vi "pinMode.vi"(3 "error in (no error)":errorcluster, 4 "Mode":enum32{"Output", "Input"}(ring), 5 "Terminal":u8, 6 "VISA Refnum in":refnum<visa-resource-name>) -> (0 "error out":errorcluster, 1 "pinMode":u8[](array[numeric]), 2 "VISA Refnum out":refnum<visa-resource-name>)   [LabVIEW 2016]
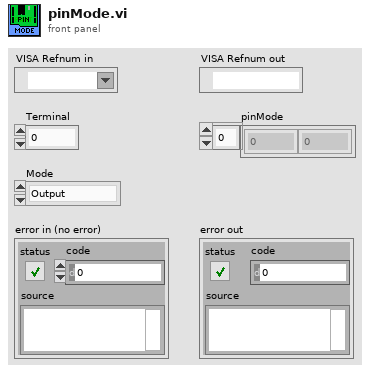
[diagram p1: front panel]
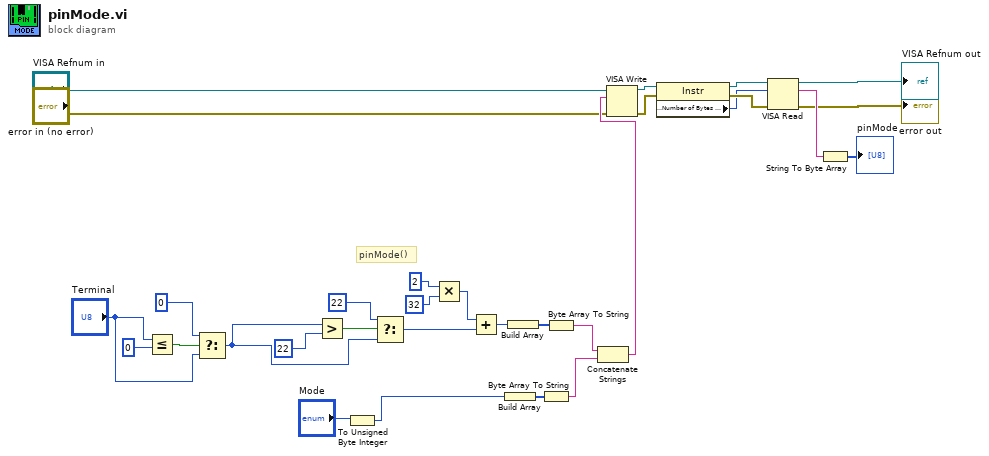
[diagram p0: block diagram]
diagram:
  # "pinMode()"
  n1 = Less Or Equal?(x="Terminal", y=u8 0) -> (x <= y?=w17:bool)
  n2 = Select(t=u8 0, s=w17, f="Terminal") -> (s? t:f=w20:u8)
  n3 = Greater?(x=w20, y=u8 22) -> (0:w12:bool)
  n4 = To Unsigned Byte Integer(number="Mode") -> (unsigned 8bit integer=w31:u8)
  n5 = Select(t=u8 22, s=w12, f=w20) -> (s? t:f=w29:u8)
  n6 = Multiply(x=u8 2, y=u8 32) -> (x*y=w15:u8)
  n7 = Add(x=w15, y=w29) -> (x+y=w21:u8)
  n8 = Build Array(w31) -> (w23:u8[])
  n9 = Build Array(w21) -> (w22:u8[])
  n10 = Byte Array To String(unsigned byte array=w23) -> (string=w24:string)
  n11 = Byte Array To String(unsigned byte array=w22) -> (string=w25:string)
  n12 = Concatenate Strings(w25, w24) -> (w26:string)
  n13 = VISA Write(VISA resource name="VISA Refnum in", write buffer=w26, error in (no error)="error in (no error)") -> (VISA resource name out=w4:refnum<visa-resource-name>, error out=w5:errorcluster)  [unwired: 1 out]
  n14 = property class="Instr"(reference=w4, error in=w5) -> (reference out=w2:refnum<visa-resource-name>, error out=w3:errorcluster, "Serial Settings:Number of Bytes at Serial Port"=w1:u32)
  n15 = VISA Read(VISA resource name=w2, byte count=w1, error in (no error)=w3) -> (VISA resource name out=→"VISA Refnum out":refnum<visa-resource-name>, read buffer=w27:string, error out=→"error out":errorcluster)  [unwired: 1 out]
  n16 = String To Byte Array(string=w27) -> (unsigned byte array=→"pinMode":u8[])
